vi "Get Create Temporary Images.vi"(8 "error in (no error)":errorcluster, 10 "Image in":T1, 11 "Analyze BaseClass in":refnum<class "Analyze BaseClass.lvclass">) -> (0 "error out":errorcluster, 1 "image mask":T1, 2 "work image":T1, 3 "Analyze BaseClass out":refnum<class "Analyze BaseClass.lvclass">, 5 "masked image":T1)   [LabVIEW 2020, in "Analyze.lvlib" / "Analyze BaseClass.lvclass"]
uses:
  Analyze BaseClass.lvclass
  <vilib>/vision/Image Controls.llb/IMAQ Image.ctl
  Analyze BaseClass.lvclass/Analyze BaseClass.ctl
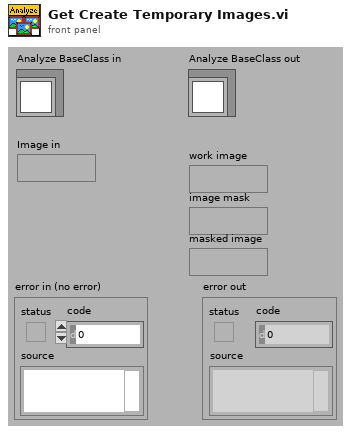
[diagram p1: front panel]
types:
  T1 = typedef "IMAQ Image.ctl" = refnum<image>
  T2 = typedef "Image Type" = u32
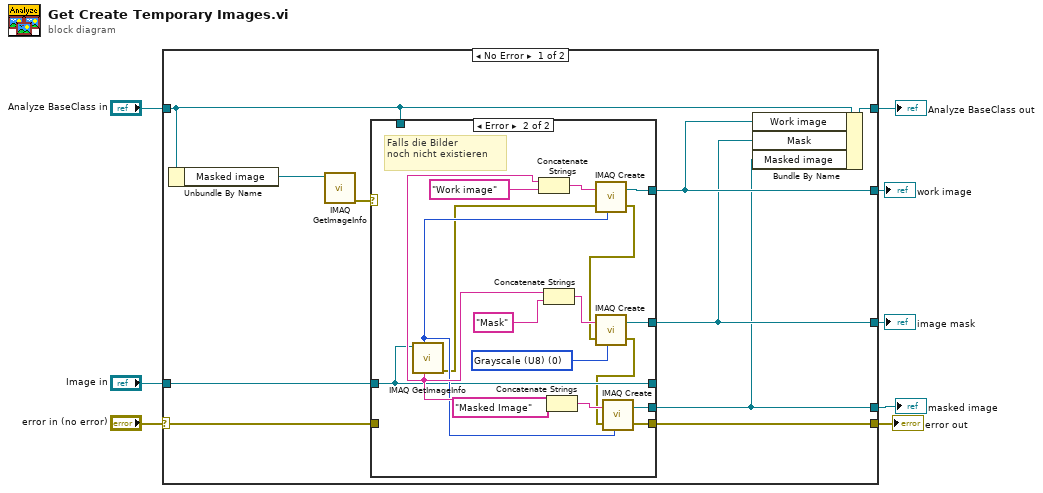
[diagram p0: block diagram]
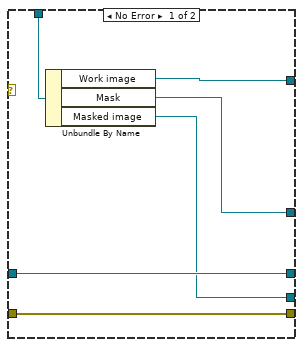
[diagram p2: hidden frame]
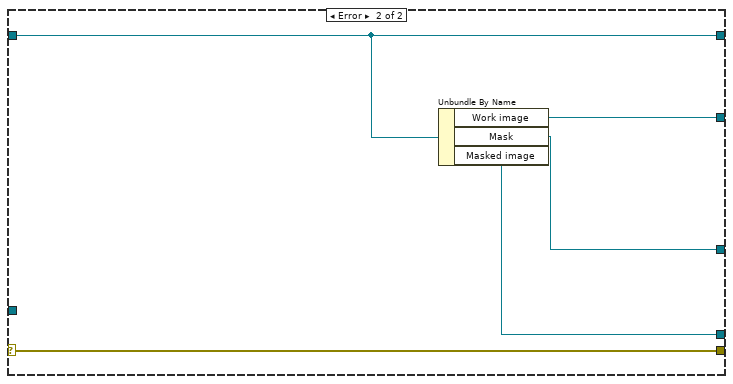
[diagram p3: hidden frame]
diagram:
  n1 = case shown="No Error" "error in (no error)" {
    selector: "error in (no error)" -> [w14 w46]
    tunnel: [w13 w46] -> w7
    tunnel: [w12 w45] -> w5
    tunnel: "Analyze BaseClass in" -> [w16 w45]
    tunnel: "Image in" -> [w15 _]
    tunnel: [w11 w44] -> w3
    tunnel: [w10 w43] -> w2
    tunnel: [w9 w42] -> w1
    frame No Error {
      n2 = Unbundle By Name(w16) -> ("Masked image"=w17:T1)
      n3 = call "IMAQ GetImageInfo"("Image"=w17) -> ("error out"=w18:errorcluster)  [unwired: 3 in, 7 out]
      n4 = case shown="Error" w18 {
        tunnel: [w22 w41] -> w11
        tunnel: [w20 w37] -> w9
        tunnel: [w21 w36] -> w10
        tunnel: w15 -> [w24 w29]
        tunnel: [w24 w29] -> _
        tunnel: [w19 w25] -> w13
        tunnel: w16 -> [w23 _]
        tunnel: w14 -> [w19 _]
        frame No Error {
          n5 = Unbundle By Name(w23) -> ("Work image"=w22:T1, "Mask"=w21:T1, "Masked image"=w20:T1)
        }
        frame Error {
          w39 = T2 0 items=["Grayscale (U8)", "Grayscale (I16)", "Grayscale (SGL)", "Complex (CSG)", "RGB (U32)", "HSL (U32)", "RGB (U64)", "Grayscale (U16)"] ("Image Type")
          # "Falls die Bilder\nnoch nicht existieren"
          n6 = call "IMAQ GetImageInfo"("Image"=w29) -> ("error out"=w28:errorcluster, "Image Name"=w31:string, "Image Type"=w30:T2)  [unwired: 3 in, 5 out]
          n7 = Concatenate Strings(w31, "Work image" ("Image Name")) -> (w35:string)
          n8 = Concatenate Strings(w31, "Mask" ("Image Name")) -> (w33:string)
          n9 = Concatenate Strings(w31, "Masked Image" ("Image Name")) -> (w32:string)
          n10 = call "IMAQ Create"("Image Name"=w35, "Image Type"=w30, "error in (no error)"=w28) -> ("New Image"=w41:T1, "error out"=w27:errorcluster)  [unwired: 2 in]
          n11 = call "IMAQ Create"("Image Name"=w33, "Image Type"=w39, "error in (no error)"=w27) -> ("New Image"=w36:T1, "error out"=w26:errorcluster)  [unwired: 2 in]
          n12 = call "IMAQ Create"("Image Name"=w32, "Image Type"=w30, "error in (no error)"=w26) -> ("New Image"=w37:T1, "error out"=w25:errorcluster)  [unwired: 2 in]
        }
      }
      n13 = Bundle By Name(cluster=w16, "Work image"=w11, "Mask"=w10, "Masked image"=w9) -> (w12:refnum<class "Analyze BaseClass.lvclass">)
    }
    frame Error {
      n14 = Unbundle By Name(w45) -> ("Work image"=w44:T1, "Mask"=w43:T1, "Masked image"=w42:T1)
    }
  }
  "error out" <- w7
  "Analyze BaseClass out" <- w5
  "work image" <- w3
  "image mask" <- w2
  "masked image" <- w1
